vi "EvaluateCompare.vi"(11 "Input":string) -> (0 "error out":errorcluster, 3 "Output":string)   [LabVIEW 2012]
uses:
  <vilib>/regexp/Match Regular Expression.xnode
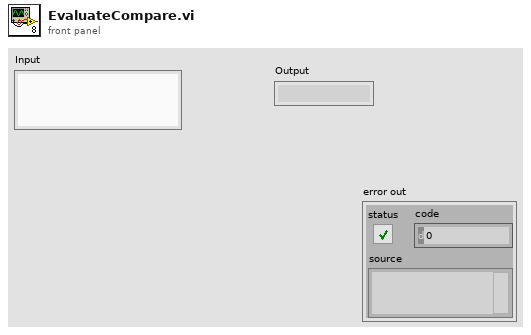
[diagram p1: front panel]
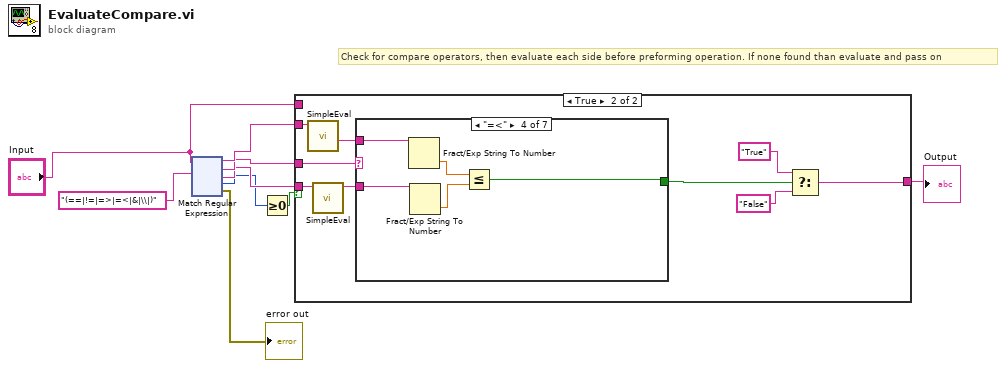
[diagram p0: block diagram]
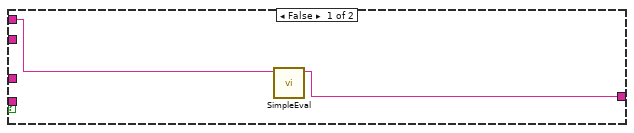
[diagram p2: hidden frame]
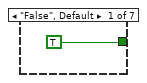
[diagram p3: hidden frame]
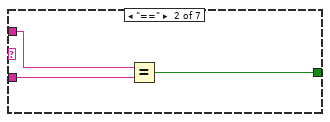
[diagram p4: hidden frame]
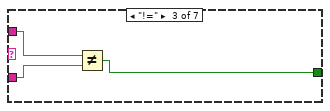
[diagram p5: hidden frame]
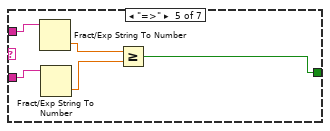
[diagram p6: hidden frame]
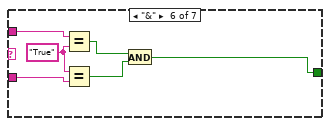
[diagram p7: hidden frame]
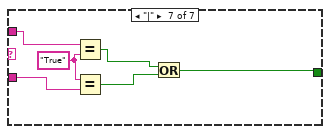
[diagram p8: hidden frame]
diagram:
  # "Check for compare operators, then evaluate each side before preforming operation. If none found than evaluate and pass on"
  n1 = xnode "Match Regular Expression"("input string"="Input", "regular expression"="(==|!=|=>|=<|&|\\|)") -> ("before match"=w6:string, "whole match"=w5:string, "after match"=w4:string, "offset past match"=w3:i32, "error out"=→"error out":errorcluster)  [unwired: 4 in]
  n2 = Greater Or Equal To 0?(x=w3) -> (x >= 0?=w1:bool)
  n3 = case shown="True" w1 {
    tunnel: [w10 w17] -> w9
    tunnel: "Input" -> [w11 _]
    tunnel: w6 -> [_ w16]
    tunnel: w5 -> [_ w15]
    tunnel: w4 -> [_ w14]
    frame False {
      n4 = call "SimpleEval.vi"("Input"=w11) -> ("Result"=w10:string)  [unwired: 10 in]
    }
    frame True {
      n5 = call "SimpleEval.vi"("Input"=w16) -> ("Result"=w20:string)  [unwired: 10 in]
      n6 = call "SimpleEval.vi"("Input"=w14) -> ("Result"=w19:string)  [unwired: 10 in]
      n7 = case shown="\"=<\"" w15 {
        tunnel: w20 -> [_ w24 w27 w31 w35 w42 w48]
        tunnel: w19 -> [_ w23 w26 w30 w36 w41 w47]
        tunnel: [TRUE w22 w25 w32 w37 w38 w44] -> w18
        frame "False", Default {
        }
        frame "==" {
          n8 = Equal?(x=w24, y=w23) -> (x = y?=w22:bool)
        }
        frame "!=" {
          n9 = Not Equal?(x=w27, y=w26) -> (x != y?=w25:bool)
        }
        frame "=<" {
          n10 = Fract/Exp String To Number(string=w31) -> (number=w28:dbl)  [unwired: 3 in, 1 out]
          n11 = Fract/Exp String To Number(string=w30) -> (number=w29:dbl)  [unwired: 3 in, 1 out]
          n12 = Less Or Equal?(x=w28, y=w29) -> (x <= y?=w32:bool)
        }
        frame "=>" {
          n13 = Fract/Exp String To Number(string=w35) -> (number=w34:dbl)  [unwired: 3 in, 1 out]
          n14 = Fract/Exp String To Number(string=w36) -> (number=w33:dbl)  [unwired: 3 in, 1 out]
          n15 = Greater Or Equal?(x=w34, y=w33) -> (x >= y?=w37:bool)
        }
        frame "&" {
          w43 = "True"
          n16 = Equal?(x=w42, y=w43) -> (x = y?=w40:bool)
          n17 = Equal?(x=w43, y=w41) -> (x = y?=w39:bool)
          n18 = And(x=w40, y=w39) -> (x .and. y?=w38:bool)
        }
        frame "|" {
          w49 = "True"
          n19 = Equal?(x=w48, y=w49) -> (x = y?=w46:bool)
          n20 = Equal?(x=w49, y=w47) -> (x = y?=w45:bool)
          n21 = Or(x=w46, y=w45) -> (x .or. y?=w44:bool)
        }
      }
      n22 = Select(t="True", s=w18, f="False") -> (s? t:f=w17:string)
    }
  }
  "Output" <- w9
